vi "EOL_FreeDiskSpace.vi"() -> ()   [LabVIEW 2017]
panel:
  in  "NewPath":path
  out "FilesArray":path[](array[path])
  in  "stop":bool
  in  "Search Button":bool
  in  "Move to Backup":bool
  out "Size":i64
  out "filenames":string[](array[string])
  in  "path":path
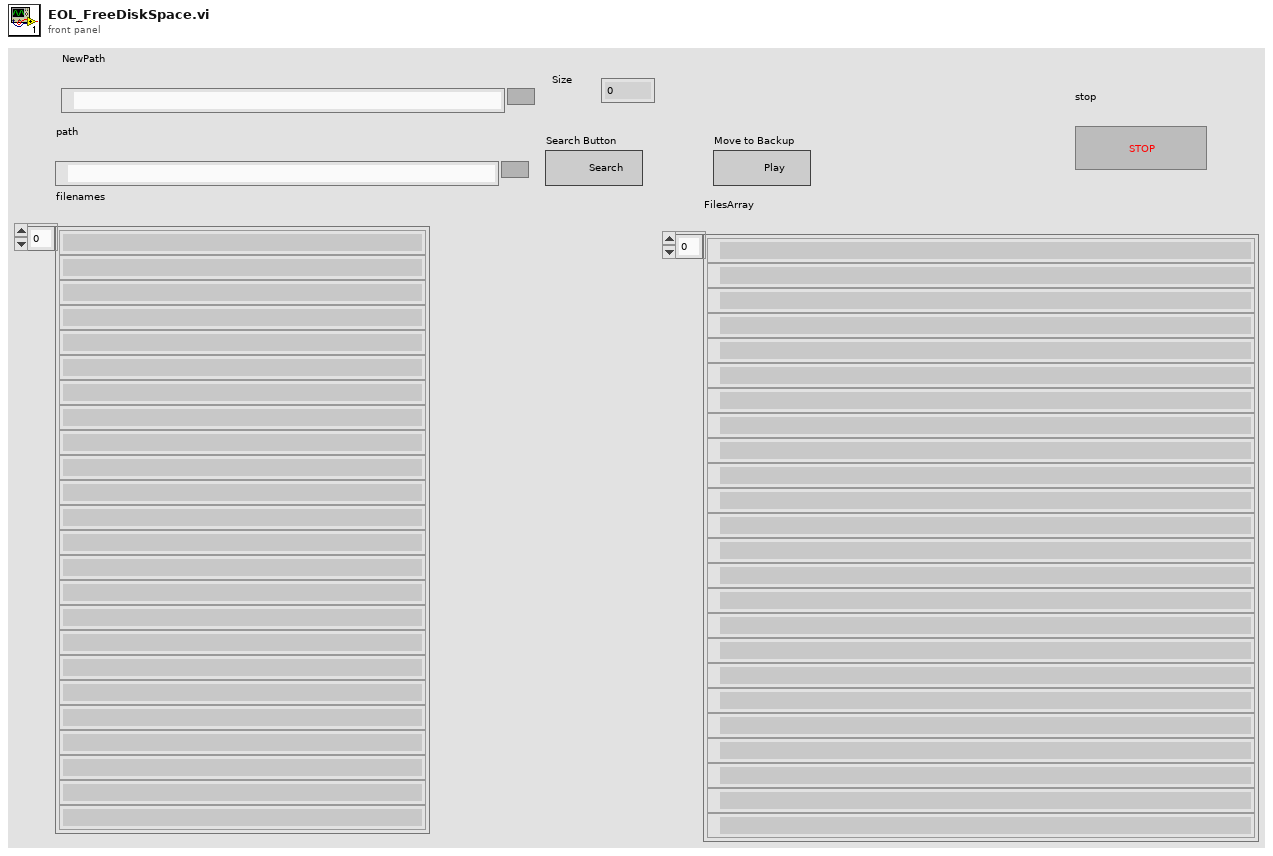
[diagram p1: front panel]
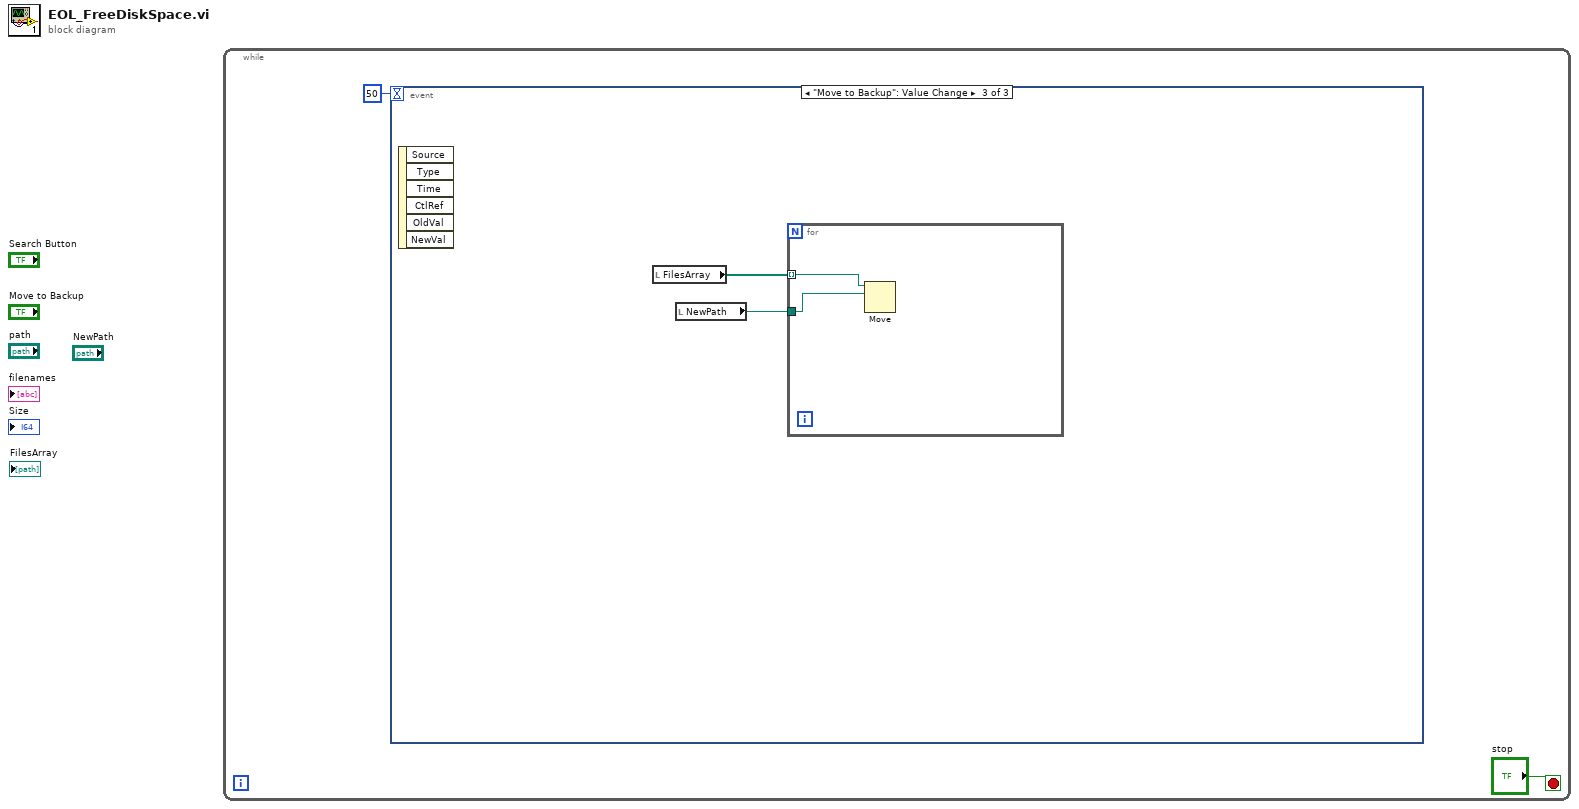
[diagram p0: block diagram]
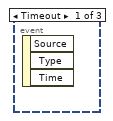
[diagram p2: hidden frame]
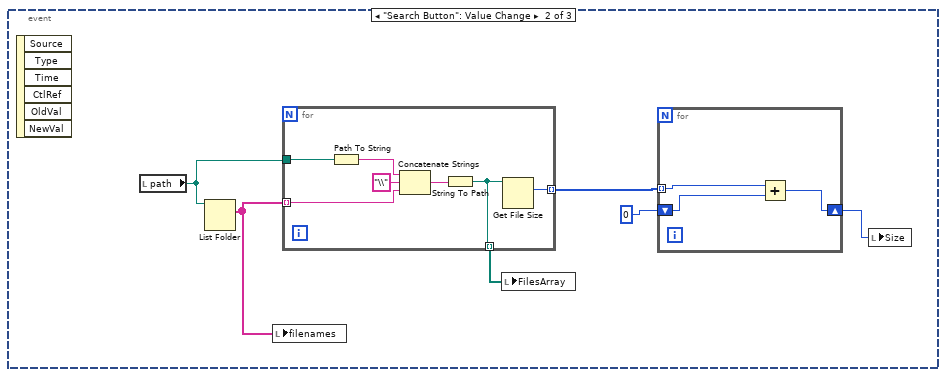
[diagram p3: hidden frame]
diagram:
  n1 = while {
    stop <- "stop" stop-if-true
    n2 = event shown="[2] \"Move to Backup\": Value Change" {
      selector: _ -> [_ _ _]
      dyn-events: _ -> [_ _ _]
      timeout: 50 -> [_ _ _]
      event Timeout {
        n3 = event-data() -> ()  [unwired: 1 in, 3 out]
      }
      event "Search Button": Value Change {
        n4 = event-data() -> ()  [unwired: 1 in, 6 out]
        n5 = local read "path"() -> (w7:path)
        n6 = List Folder(path=w7) -> (filenames=w6:string[])  [unwired: 3 in, 3 out]
        n7 = local write "filenames"(w6) -> ()
        n8 = for {
          tunnel: w6 -> [w15] mode=indexing
          tunnel: w7 -> [w18]
          tunnel: [w13] -> w4 mode=indexing
          tunnel: [w12] -> w3 mode=indexing
          n9 = Path To String(path=w18) -> (string=w17:string)
          n10 = Concatenate Strings(w17, "\\" ("string"), w15) -> (w14:string)
          n11 = String To Path(string=w14) -> (path=w12:path)
          n12 = Get File Size(file=w12) -> (size (in bytes)=w13:i64)  [unwired: 1 in, 2 out]
        }
        n13 = local write "FilesArray"(w3) -> ()
        n14 = for {
          tunnel: w4 -> [w10] mode=indexing
          shift-right: [w9] -> w5
          shift-left: 0 -> [w11]
          n15 = Add(x=w10, y=w11) -> (x+y=w9:i64)
        }
        n16 = local write "Size"(w5) -> ()
      }
      event "Move to Backup": Value Change {
        n17 = event-data() -> ()  [unwired: 1 in, 6 out]
        n18 = local read "FilesArray"() -> (w20:path[])
        n19 = local read "NewPath"() -> (w19:path)
        n20 = for {
          tunnel: w20 -> [w22] mode=indexing
          tunnel: w19 -> [w21]
          n21 = Move(source path=w22, 10:w21) -> ()  [unwired: 3 in, 3 out]
        }
      }
    }
  }
